vi "PSDAQ_DATA_View All Queue Date.vi"(8 "error in (no error)":errorcluster, 10 "Index":i32[](array[numeric]), 11 "Queue Datas":string[][](array[string])) -> (0 "error out":errorcluster, 1 "Update?":bool, 2 "Index Out":i32[](array[numeric]), 3 "Queue Data":T1)   [LabVIEW 2016]
uses:
  Q-View.vi
  PSDAQEG_Task Queue Type.ctl
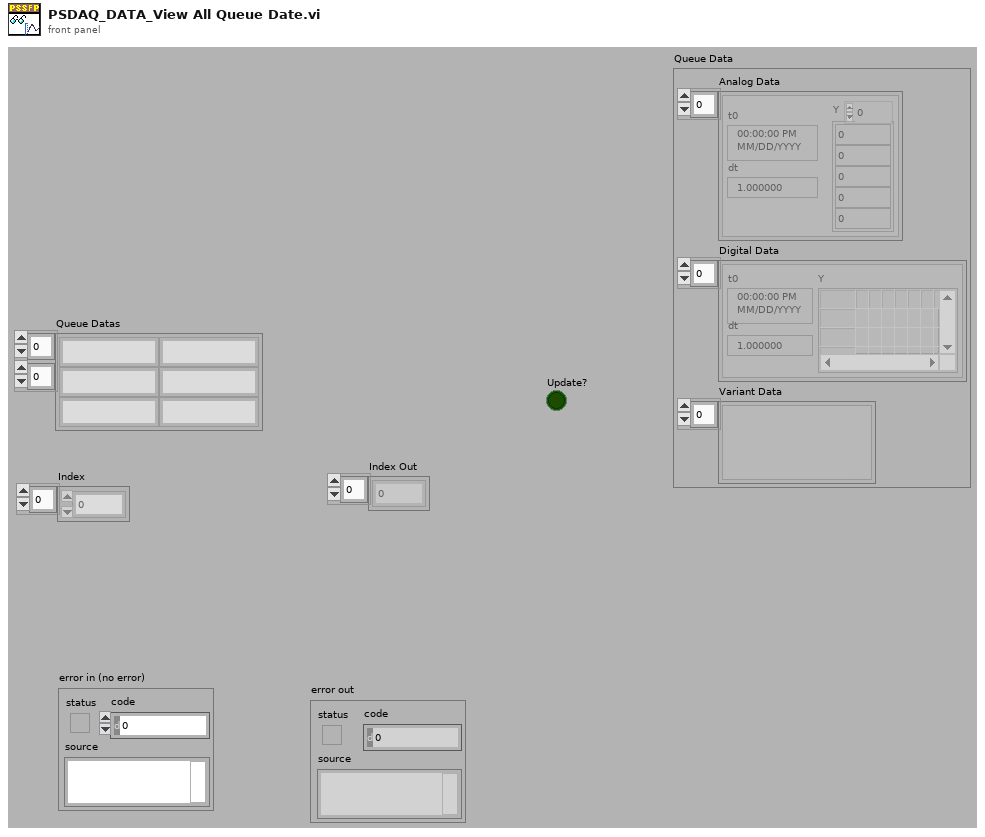
[diagram p1: front panel]
types:
  T1 = cluster{"Analog Data":waveform(dbl)[], "Digital Data":digitalwaveform[], "Variant Data":variant[]}
  T2 = typedef "PSDAQEG_Task Queue Type.ctl" = enum16{"Analog", "Digital", "Variant"}
  T3 = cluster{"Index":i32, "Waveform":waveform(dbl)[]}[]
  T4 = cluster{"max queue size (-1, unlimited)":i32, digitalwaveform[]}[]
  T5 = cluster{"max queue size (-1, unlimited)":i32, variant[]}[]
  T6 = cluster{"max queue size (-1, unlimited)":i32, digitalwaveform[]}
  T7 = cluster{"max queue size (-1, unlimited)":i32, variant[]}
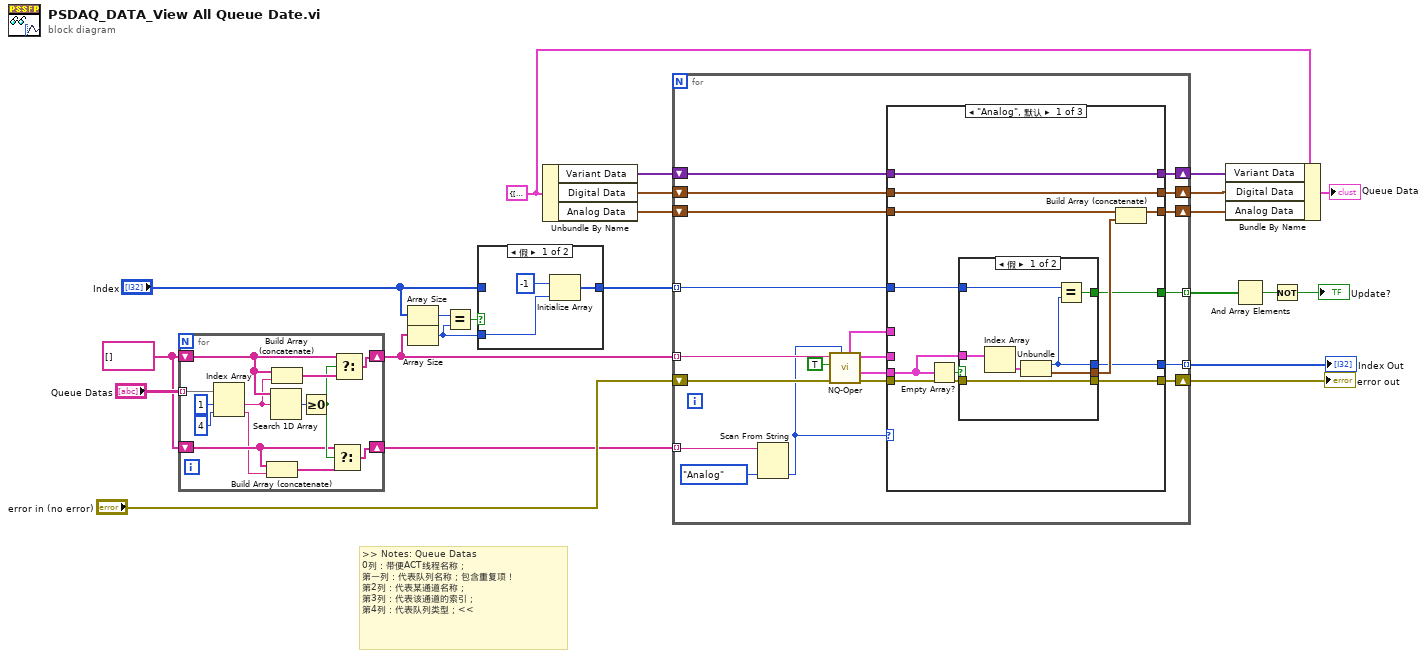
[diagram p0: block diagram]
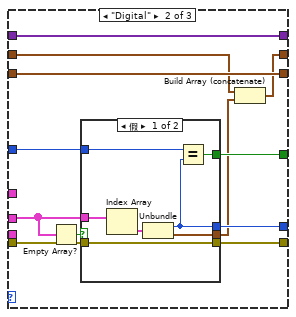
[diagram p3: hidden frame]
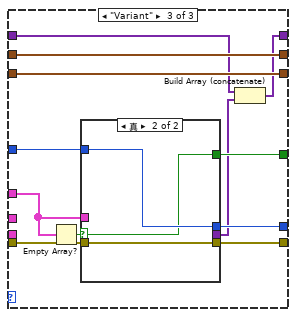
[diagram p5: hidden frame]
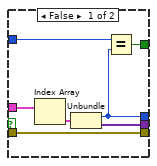
[diagram p6: hidden frame]
diagram:
  w5 = T1 {"Analog Data"=[], "Digital Data"=[], "Variant Data"=[]} ("Read Data")
  w11 = string[] []
  # ">> Notes: Queue Datas\n0列：带便ACT线程名称；\n第一列：代表队列名称；包含重复项！\n第2列：代表某通道名称；\n第3列：代表该通道的索引；\n第4列：代表队列类型；<<"
  n1 = for {
    tunnel: "Queue Datas" -> [w36] mode=indexing
    shift-right: [w30] -> w23
    shift-left: w11 -> [w33]
    shift-right: [w28] -> w10
    shift-left: w11 -> [w26]
    n2 = Index Array(array=w36, index #1=1 ("index"), index #2=4 ("index")) -> (element #1=w32:string, element #2=w25:string)
    n3 = Build Array (concatenate)(w26, w25) -> (w24:string[])
    n4 = Search 1D Array(1D array=w33, element=w32) -> (index of element=w34:i32)  [unwired: 1 in]
    n5 = Build Array (concatenate)(w33, w32) -> (w31:string[])
    n6 = Greater Or Equal To 0?(x=w34) -> (x >= 0?=w27:bool)
    n7 = Select(t=w26, s=w27, f=w24) -> (s? t:f=w28:string[])
    n8 = Select(t=w33, s=w27, f=w31) -> (s? t:f=w30:string[])
  }
  n9 = Array Size(array="Index") -> (size(s)=w22:i32)
  n10 = Array Size(array=w23) -> (size(s)=w20:i32)
  n11 = Equal?(x=w22, y=w20) -> (x = y?=w21:bool)
  n12 = case shown="假" w21 {
    tunnel: [w37 w40] -> w19
    tunnel: "Index" -> [_ w40]
    tunnel: w20 -> [w39 _]
    frame False {
      n13 = Initialize Array(-1, w39) -> (w37:i32[])
    }
    frame True {
    }
  }
  n14 = Unbundle By Name(w5) -> ("Variant Data"=w7:variant[], "Digital Data"=w8:digitalwaveform[], "Analog Data"=w9:waveform(dbl)[])
  n15 = for {
    tunnel: w23 -> [w58] mode=indexing
    shift-right: [w59] -> w2
    shift-left: w9 -> [w60]
    tunnel: w19 -> [w55] mode=indexing
    tunnel: [w54] -> w16 mode=indexing
    tunnel: [w53] -> w18 mode=indexing
    shift-right: [w52] -> w13
    shift-left: "error in (no error)" -> [w51]
    tunnel: w10 -> [w49] mode=indexing
    shift-right: [w43] -> w3
    shift-left: w8 -> [w44]
    shift-right: [w41] -> w4
    shift-left: w7 -> [w42]
    n16 = Scan From String(input string=w49, default 1=PSDAQEG_Task_Queue_Type."Analog" ("Queue Type")) -> (output 1=w48:T2)  [unwired: 3 in, 3 out]
    n17 = call-poly "NQ-Oper.vi"("Queue Type"=w48, "error in"=w51, "Return Elements? (F)"=TRUE ("Return Elements?(F)"), "Q Name"=w58) -> ("error out"=w57:errorcluster, "Analog data"=w47:T3, "Digital Data"=w46:T4, "Variant Data"=w45:T5)  [unwired: 3 in, 1 out]
    n18 = case shown="\"Analog\", 默认" w48 {
      tunnel: w60 -> [w70 w88 w110]
      tunnel: [w69 w88 w110] -> w59
      tunnel: w57 -> [w68 w93 w115]
      tunnel: w55 -> [w67 w92 w114]
      tunnel: [w66 w91 w113] -> w54
      tunnel: [w65 w90 w112] -> w53
      tunnel: [w64 w89 w111] -> w52
      tunnel: w47 -> [w63 _ _]
      tunnel: w46 -> [_ w87 _]
      tunnel: w45 -> [_ _ w108]
      tunnel: w44 -> [w62 w85 w109]
      tunnel: [w62 w84 w109] -> w43
      tunnel: w42 -> [w61 w83 w106]
      tunnel: [w61 w83 w105] -> w41
      frame "Analog", Default {
        n19 = Empty Array?(array=w63) -> (empty?=w72:bool)
        n20 = case shown="假" w72 {
          selector: w72 -> [_ w81]
          tunnel: w63 -> [w79 _]
          tunnel: w68 -> [w73 w80]
          tunnel: [w75 _] -> w71
          tunnel: w67 -> [w77 w82]
          tunnel: [w76 w82] -> w66
          tunnel: [w74 w81] -> w65
          tunnel: [w73 w80] -> w64
          frame False {
            n21 = Index Array(array=w79) -> (element=w78:cluster{"Index":i32, "Waveform":waveform(dbl)[]})  [unwired: 1 in]
            n22 = Unbundle(w78) -> ("Index"=w76:i32, "Waveform"=w75:waveform(dbl)[])
            n23 = Equal?(x=w77, y=w76) -> (x = y?=w74:bool)
          }
          frame True {
          }
        }
        n24 = Build Array (concatenate)(w70, w71) -> (w69:waveform(dbl)[])
      }
      frame "Digital" {
        n25 = Empty Array?(array=w87) -> (empty?=w94:bool)
        n26 = case shown="假" w94 {
          selector: w94 -> [_ w103]
          tunnel: w87 -> [w101 _]
          tunnel: w93 -> [w95 w102]
          tunnel: [w97 _] -> w86
          tunnel: w92 -> [w99 w104]
          tunnel: [w98 w104] -> w91
          tunnel: [w96 w103] -> w90
          tunnel: [w95 w102] -> w89
          frame False {
            n27 = Index Array(array=w101) -> (element=w100:T6)  [unwired: 1 in]
            n28 = Unbundle(w100) -> ("max queue size (-1, unlimited)"=w98:i32, w97:digitalwaveform[])
            n29 = Equal?(x=w99, y=w98) -> (x = y?=w96:bool)
          }
          frame True {
          }
        }
        n30 = Build Array (concatenate)(w85, w86) -> (w84:digitalwaveform[])
      }
      frame "Variant" {
        n31 = Empty Array?(array=w108) -> (empty?=w116:bool)
        n32 = case shown="真" w116 {
          selector: w116 -> [_ w125]
          tunnel: w108 -> [w123 _]
          tunnel: w115 -> [w117 w124]
          tunnel: [w119 _] -> w107
          tunnel: w114 -> [w121 w126]
          tunnel: [w120 w126] -> w113
          tunnel: [w118 w125] -> w112
          tunnel: [w117 w124] -> w111
          frame False {
            n33 = Index Array(array=w123) -> (element=w122:T7)  [unwired: 1 in]
            n34 = Unbundle(w122) -> ("max queue size (-1, unlimited)"=w120:i32, w119:variant[])
            n35 = Equal?(x=w121, y=w120) -> (x = y?=w118:bool)
          }
          frame True {
          }
        }
        n36 = Build Array (concatenate)(w106, w107) -> (w105:variant[])
      }
    }
  }
  "Index Out" <- w16
  "error out" <- w13
  n37 = Bundle By Name(cluster=w5, "Variant Data"=w4, "Digital Data"=w3, "Analog Data"=w2) -> (→"Queue Data":T1)
  n38 = And Array Elements(Boolean array=w18) -> (logical AND=w6:bool)
  n39 = Not(x=w6) -> (.not. x?=→"Update?":bool)
